vi "获取更新信息.vi"(8 "error in (no error)":errorcluster caption="错误输入（无错误）") -> (0 "error out":errorcluster caption="错误输出", 3 "更新文件路径":path)   [LabVIEW 2017]
uses:
  <vilib>/Utility/config.llb/Read Key (String).vi
  <vilib>/Utility/config.llb/Read Key (I32).vi
  <vilib>/Utility/config.llb/NI_LVConfig.lvlib
  <vilib>/FTP/NI_FTP.lvlib
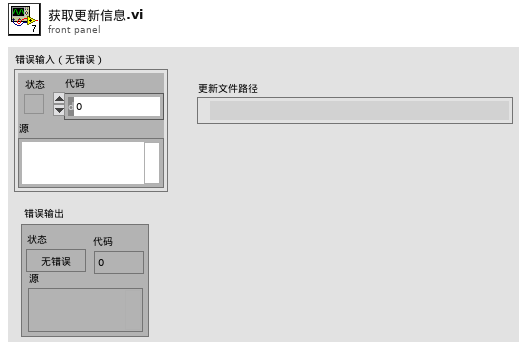
[diagram p1: front panel]
types:
  T1 = typedef "NI_LVConfig.lvlib/Config Data RefNum.ctl" = refnum<k1>
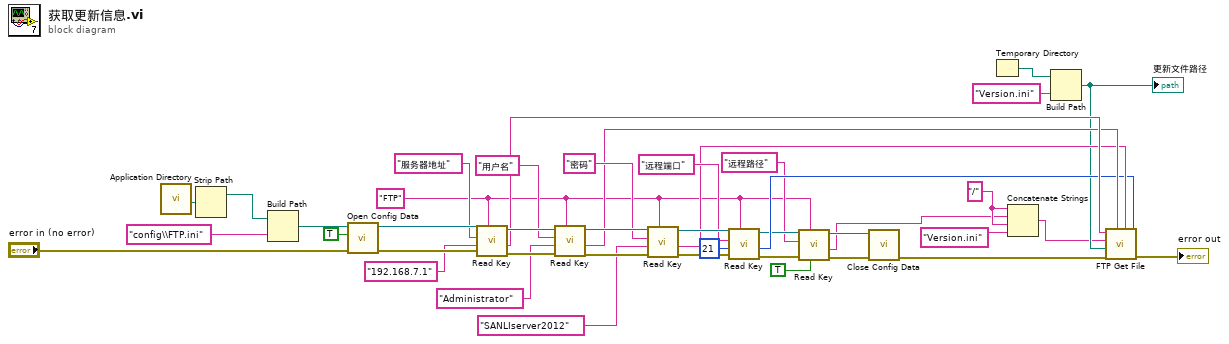
[diagram p0: block diagram]
diagram:
  w8 = "/" ("字符串")
  w7 = "FTP" ("section")
  n1 = call <vilib>:"Application Directory.vi"() -> ("Application Directory"=w2:path)
  n2 = Strip Path(path=w2) -> (stripped path=w1:path)  [unwired: 1 out]
  n3 = Build Path(base path=w1, name or relative path="config\\FTP.ini" ("名称或相对路径")) -> (appended path=w36:path)
  n4 = call <vilib>:"Open Config Data.vi"("error in (no error)"="error in (no error)", "create file if necessary (T)"=TRUE, "configuration file path"=w36) -> ("error out"=w42:errorcluster, "refnum"=w37:T1)  [unwired: 6 in, 1 out]
  n5 = call-poly <vilib>:"Read Key.vi"("section"=w7, "error in (no error)"=w42, "default value"="192.168.7.1", "key"="服务器地址", "refnum"=w37) -> ("error out"=w41:errorcluster, "value"=w22:string, "refnum out"=w38:T1)  [unwired: 3 in, 1 out]
  n6 = call-poly <vilib>:"Read Key.vi"("section"=w7, "error in (no error)"=w41, "default value"="Administrator", "key"="用户名", "refnum"=w38) -> ("error out"=w40:errorcluster, "value"=w21:string, "refnum out"=w39:T1)  [unwired: 3 in, 1 out]
  n7 = call-poly <vilib>:"Read Key.vi"("section"=w7, "error in (no error)"=w40, "default value"="SANLIserver2012", "key"="密码", "refnum"=w39) -> ("error out"=w28:errorcluster, "value"=w20:string, "refnum out"=w27:T1)  [unwired: 3 in, 1 out]
  n8 = call-poly <vilib>:"Read Key.vi"("section"=w7, "error in (no error)"=w28, "default value"=21, "key"="远程端口", "refnum"=w27) -> ("error out"=w18:errorcluster, "value"=w19:i32, "refnum out"=w15:T1)  [unwired: 3 in, 1 out]
  n9 = call-poly <vilib>:"Read Key.vi"("read raw string? (F)"=TRUE, "section"=w7, "error in (no error)"=w18, "key"="远程路径", "refnum"=w15) -> ("error out"=w17:errorcluster, "value"=w3:string, "refnum out"=w16:T1)  [unwired: 3 in, 1 out]
  n10 = call <vilib>:"Close Config Data.vi"("error in (no error)"=w17, "refnum"=w16) -> ("error out"=w23:errorcluster)  [unwired: 8 in, 1 out]
  n11 = Temporary Directory() -> (w13:path)
  n12 = Concatenate Strings(w8, w3, w8, "Version.ini" ("字符串")) -> (w5:string)
  n13 = Build Path(base path=w13, name or relative path="Version.ini" ("名称或相对路径")) -> (appended path=w11:path)
  "更新文件路径" <- w11
  n14 = call <vilib>:"FTP Get File.vi"("remote port (21)"=w19, "password"=w20, "user"=w21, "error in (no error)"=w23, "local path"=w11, "remote path"=w5, "host"=w22) -> ("error out"=→"error out":errorcluster)  [unwired: 3 in, 1 out]
